vi "Analyze Doppler waveforms v2.vi"() -> ()   [LabVIEW 2022 SP3]
uses:
  Instance           5 36Saved   Analyze Doppler waveforms v2 .vi
  Instance           6 36Saved   Analyze Doppler waveforms v2 .vi
  Instance           4 36Saved   Analyze Doppler waveforms v2 .vi
  Instance           3 36Saved   Analyze Doppler waveforms v2 .vi
  <vilib>/gmath/NI_Gmath.lvlib
  <vilib>/Analysis/NI_AALPro.lvlib
panel:
  out "number of peaks":i32
  in  "threshold":dbl
  out "threshold peaks indices":i32[](array[numeric])
  in  "pres to get <f>":bool
  out "Array 2":dbl[](array[numeric])
  out "Waveform Graph 3":dbl[](graph)
  out "Number of samples 2":i32
  out "average frequency":dbl
  out "frequency profile":dbl[](graph)
  out "Waveform Graph":dynamicdata(graph)
  out "Waveform Graph 2":dbl[](graph)
  in  "stop":bool
  in  "Boolean":bool
  out "Array":dbl[](array[numeric])
  out "Spectrogram":dbl[][](graph)
  out "Number of samples":i32
  in  "Frame time shift":i32(slide)=32 caption="in mumber of samples" min=4 max=512 step=2 scale=0.0..512.0
  out "Sampling frequency":dbl
  in  "window selector":i32(ring)=4 format="%0.0f" items=["Rectangular", "Blackman", "Hamming", "Hanning", "Gaussian"]
  in  "Frame width":i32(slide)=128 min=2 max=1024 step=2 scale=0.0..1024.0
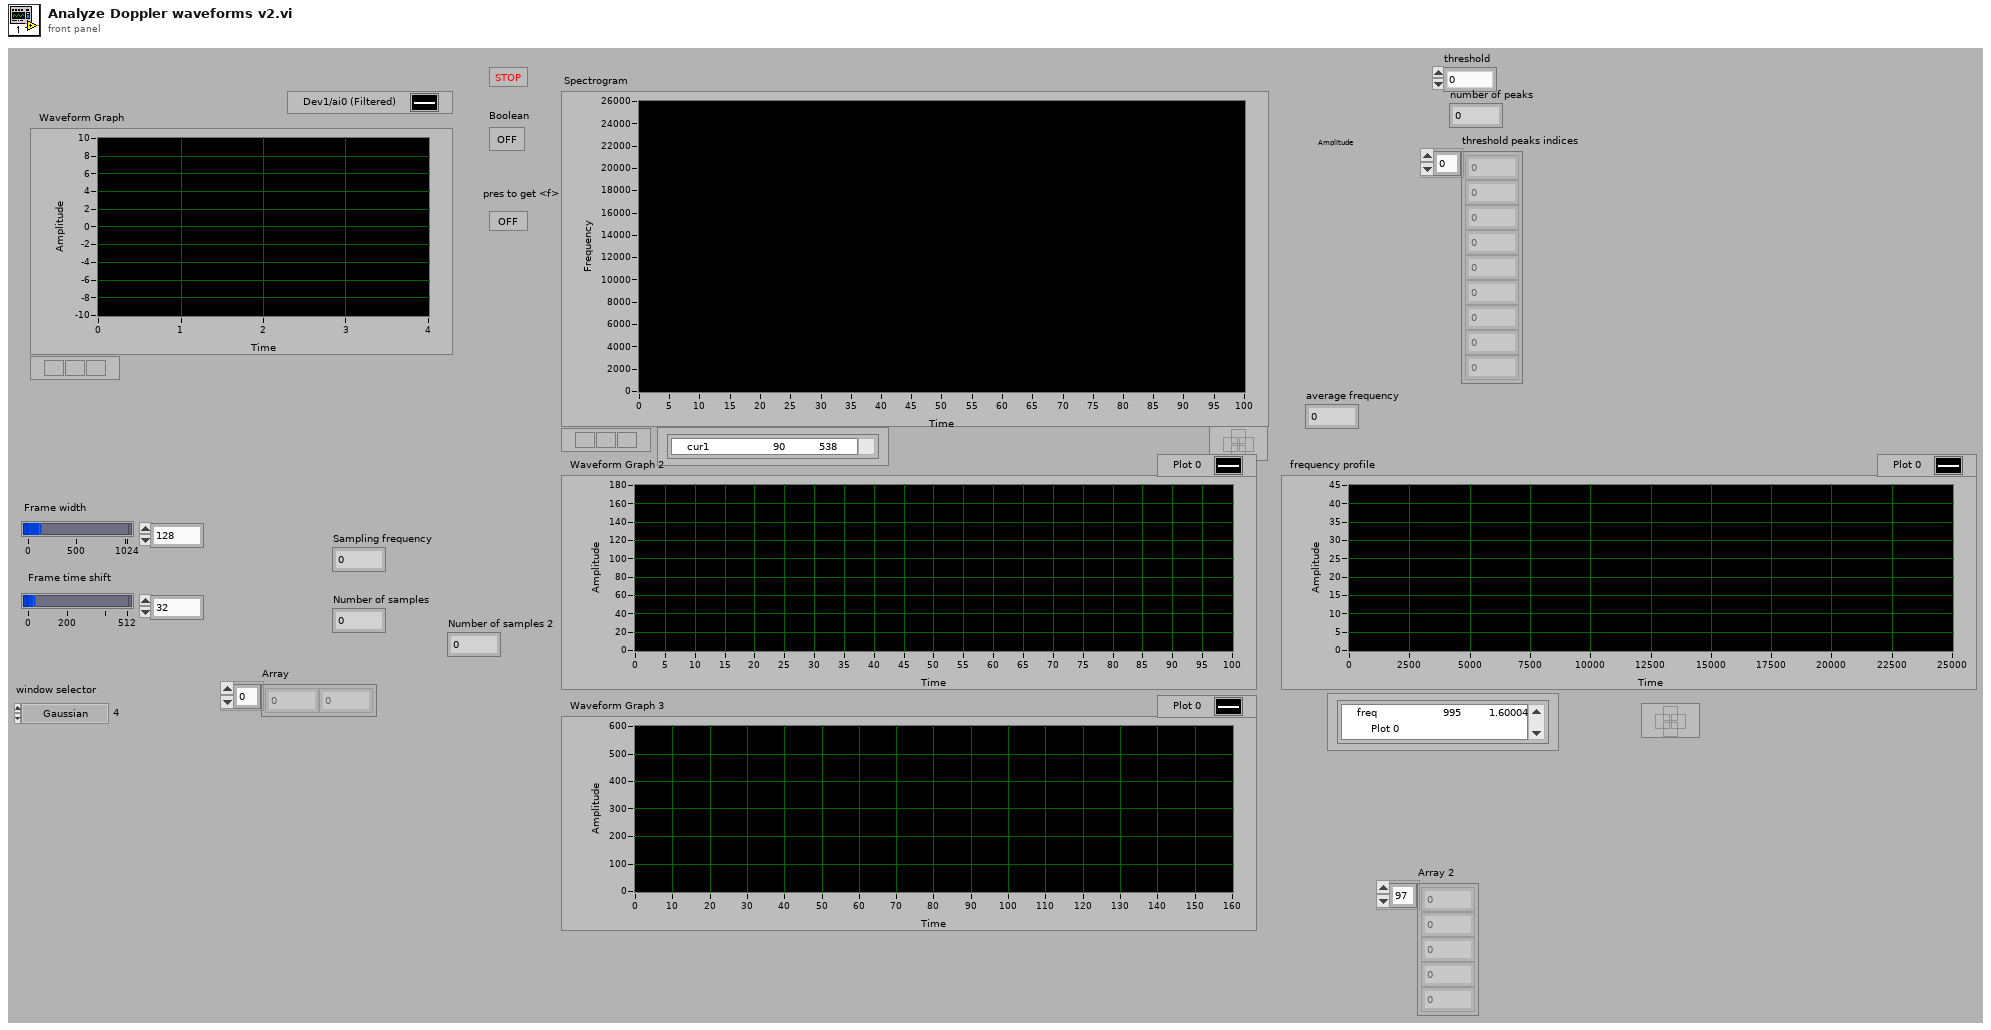
[diagram p1: front panel]
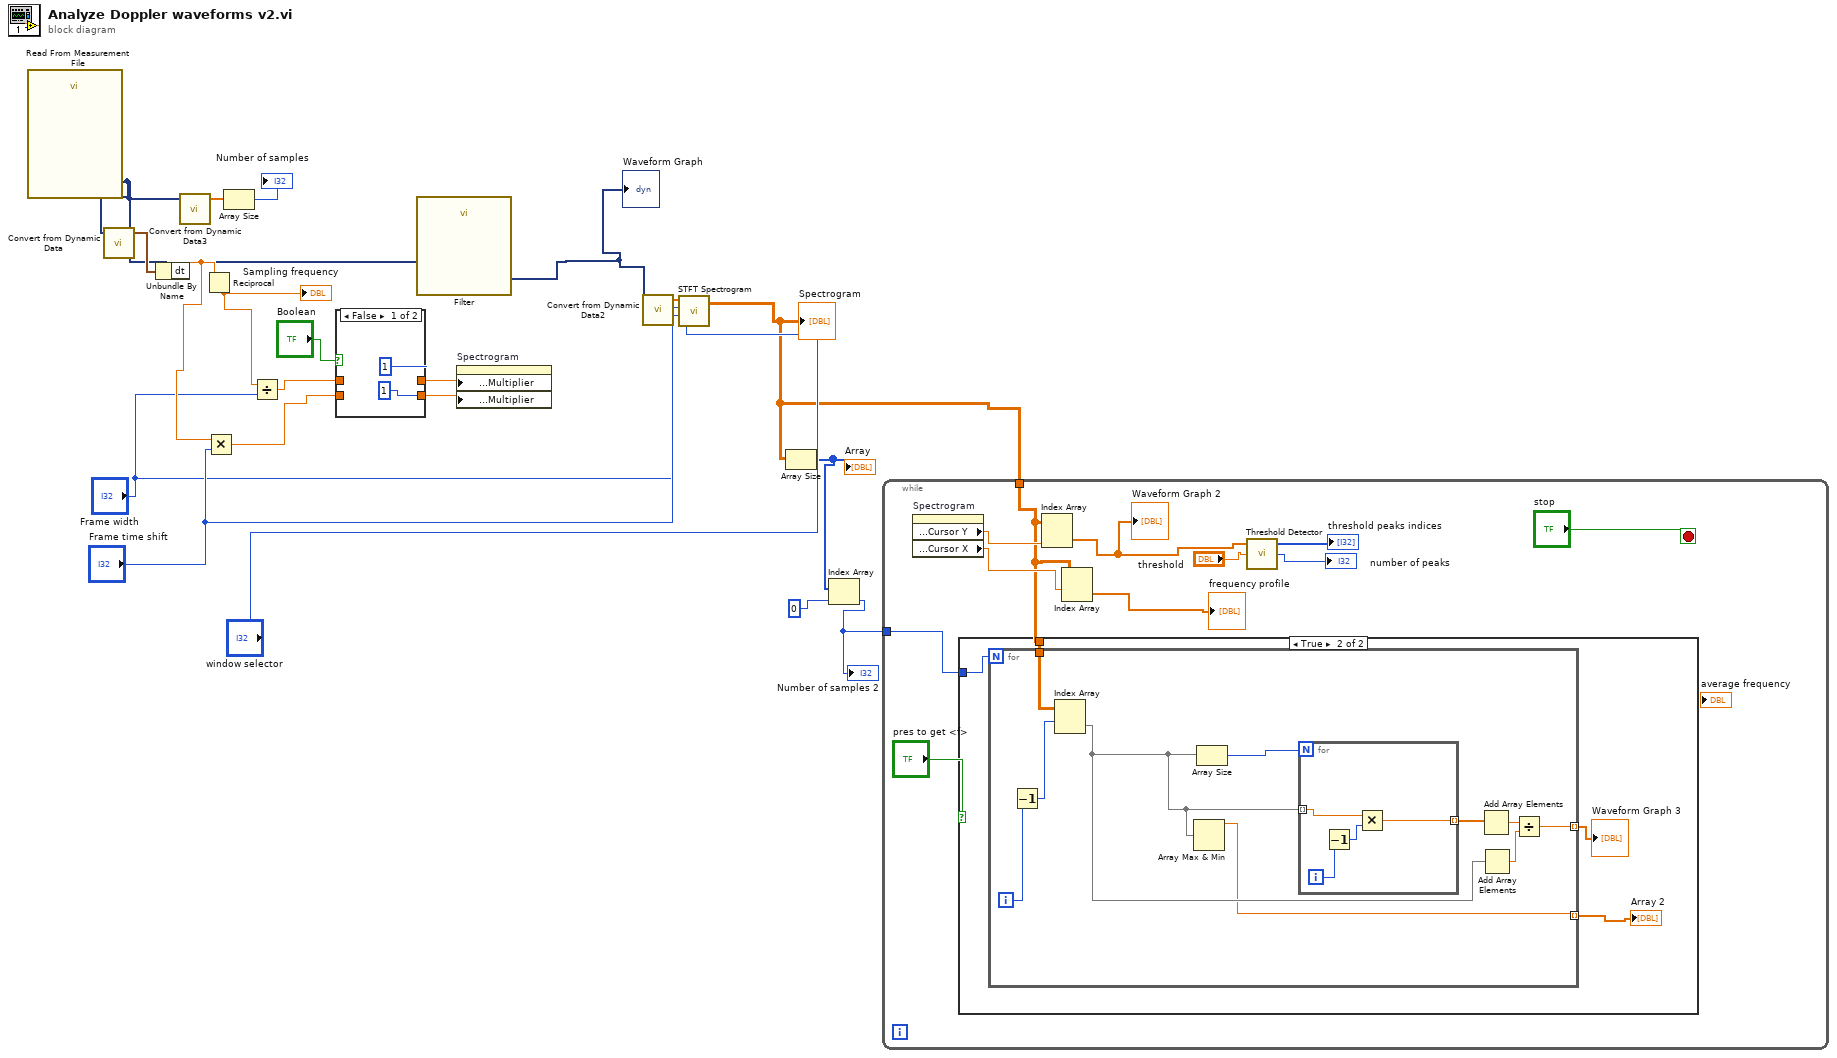
[diagram p0: block diagram]
diagram:
  n1 = call "Read From Measurement File"() -> ("Signals"=w11:dynamicdata)  [unwired: 4 in, 7 out]
  n2 = call "Convert from Dynamic Data"("Dynamic Data Type"=w11) -> ("Waveform"=w20:waveform(dbl))  [unwired: 1 in, 2 out]
  n3 = Unbundle By Name(w20) -> ("dt"=w17:dbl)
  n4 = call "Convert from Dynamic Data3"("Dynamic Data Type"=w11) -> ("Array"=w19:dbl[])  [unwired: 3 out]
  n5 = Reciprocal(x=w17) -> (1/x=w18:dbl)
  "Sampling frequency" <- w18
  n6 = Multiply(x=w17, y="Frame time shift") -> (x*y=w16:dbl)
  n7 = Array Size(array=w19) -> (size(s)=→"Number of samples":i32)
  n8 = Divide(x=w18, y="Frame width") -> (x/y=w10:dbl)
  n9 = case shown="False" "Boolean" {
    tunnel: w16 -> [_ w23]
    tunnel: w10 -> [_ w24]
    tunnel: [1 w24] -> w8
    tunnel: [1 w23] -> w7
    frame False {
    }
    frame True {
    }
  }
  n10 = call "Filter"("Signal"=w11) -> ("Filtered Signal"=w5:dynamicdata)  [unwired: 2 in, 8 out]
  "Waveform Graph" <- w5
  n11 = property on="Spectrogram" class="IntGraph (strict)"("Y Scale.Offset and Multiplier:Multiplier"=w8, "X Scale.Offset and Multiplier:Multiplier"=w7) -> ()  [unwired: 2 in, 2 out]
  n12 = call "Convert from Dynamic Data2"("Dynamic Data Type"=w5) -> ("Array"=w4:dbl[])  [unwired: 3 out]
  n13 = call <vilib>:"STFT Spectrogram.vi"("window selector"="window selector", "window length"="Frame width", "time increment"="Frame time shift", "X"=w4) -> ("STFT Spectrogram {X}"=w6:dbl[][])  [unwired: 1 out]
  "Spectrogram" <- w6
  n14 = Array Size(array=w6) -> (size(s)=w3:i32[])
  "Array" <- w3
  n15 = Index Array(array=w3, index=0) -> (element=w1:i32)
  "Number of samples 2" <- w1
  n16 = while {
    tunnel: w6 -> [w26]
    tunnel: w1 -> [w34]
    stop <- "stop" stop-if-true
    n17 = property on="Spectrogram" class="IntGraph (strict)"() -> ("Cursor.Cursor Position:Cursor Y"=w35:dbl, "Cursor.Cursor Position:Cursor X"=w27:dbl)  [unwired: 2 in, 2 out]
    n18 = case shown="True" "pres to get <f>" {
      tunnel: w26 -> [_ w39]
      tunnel: w34 -> [_ w38]
      frame False {
      }
      frame True {
        n19 = for {
          N: w38 -> [_]
          tunnel: w39 -> [w49]
          tunnel: [w44] -> w37 mode=indexing
          tunnel: [w40] -> w36 mode=indexing
          i -> [w43]
          n20 = Decrement(x=w43) -> (x-1=w42:i32)
          n21 = Index Array(array=w49, index (row)=w42) -> (element=w41:dbl[])  [unwired: 1 in]
          n22 = Array Max & Min(array=w41) -> (max value=w40:dbl)  [unwired: 3 out]
          n23 = Array Size(array=w41) -> (size(s)=w48:i32)
          n24 = for {
            N: w48 -> [_]
            tunnel: w41 -> [w51] mode=indexing
            tunnel: [w50] -> w47 mode=indexing
            i -> [w52]
            n25 = Decrement(x=w52) -> (x-1=w53:i32)
            n26 = Multiply(x=w51, y=w53) -> (x*y=w50:dbl)
          }
          n27 = Add Array Elements(numeric array=w47) -> (sum=w46:dbl)
          n28 = Add Array Elements(numeric array=w41) -> (sum=w45:dbl)
          n29 = Divide(x=w46, y=w45) -> (x/y=w44:dbl)
        }
        "Waveform Graph 3" <- w37
        "Array 2" <- w36
      }
    }
    n30 = Index Array(array=w26, index (col)=w35) -> (element=w32:dbl[])  [unwired: 1 in]
    "Waveform Graph 2" <- w32
    n31 = Index Array(array=w26, index (row)=w27) -> (element=→"frequency profile":dbl[])  [unwired: 1 in]
    n32 = call <vilib>:"Threshold Detector.vi"("threshold"="threshold", "X"=w32) -> ("count"=→"number of peaks":i32, "Indices"=→"threshold peaks indices":i32[])  [unwired: 1 in, 1 out]
  }
